vi "PC Code 2.vi"() -> ()   [LabVIEW 2014]
uses:
  <vilib>/Instr/_visa.llb/VISA Flush IO Buffer Mask.ctl
panel:
  in  "stop":bool caption="ESTOP"
  out "String Received":string
  in  "VISA resource name":refnum<visa-resource-name>="COM10"
  in  "error in":errorcluster
  out "Battery\nVolts":i16
  out "Mode":i16=1
  out "Local\nHeading":i16=90
  out "Desired \nVelocity":i16=5
  out "Dist":i16
  out "IR Index":i32
  out "error out":errorcluster
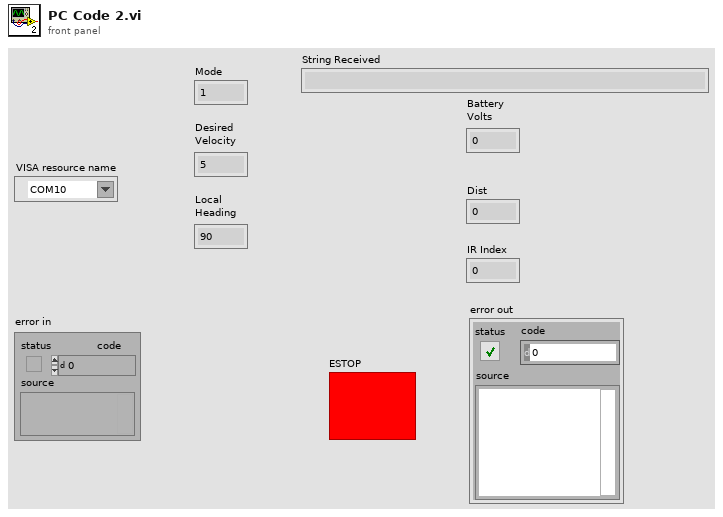
[diagram p1: front panel]
types:
  T1 = typedef "VISA Flush IO Buffer Mask.ctl" = u16
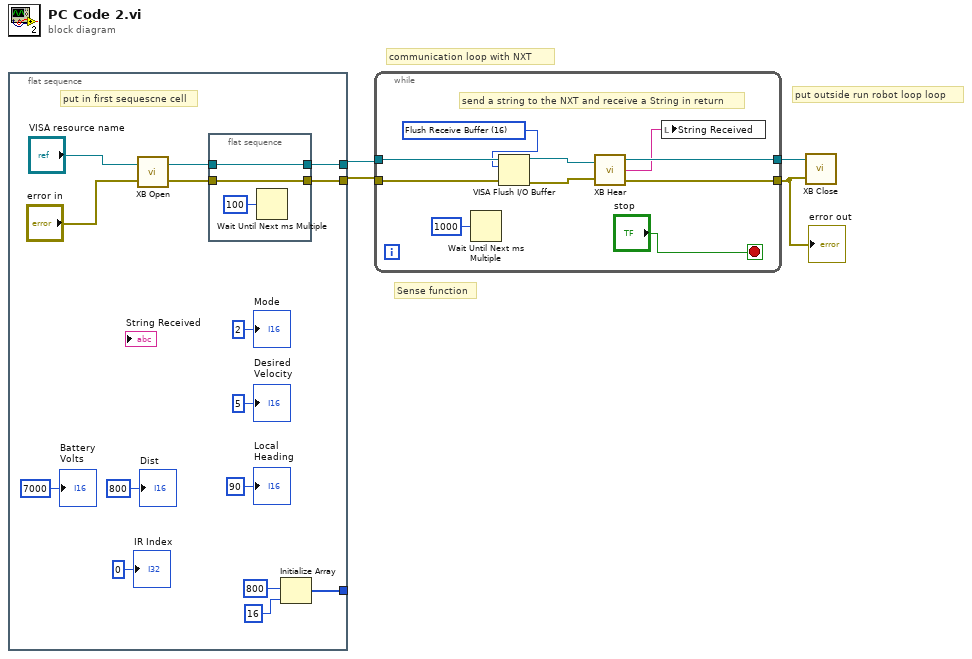
[diagram p0: block diagram]
diagram:
  # "put outside run robot loop loop"
  # "Sense function"
  # "communication loop with NXT"
  n1 = flat-sequence {
    tunnel: [w15] -> w3
    tunnel: [w14] -> w2
    tunnel: [w5] -> _
    frame #0 {
      # "put in first sequescne cell"
      n2 = call "XB Open.vi"("error in (no error)"="error in", "VISA resource name"="VISA resource name") -> ("error out"=w18:errorcluster, "VISA resource name out"=w19:refnum<visa-resource-name>)
      n3 = flat-sequence {
        tunnel: w19 -> [w20]
        tunnel: w18 -> [w21]
        tunnel: [w21] -> w14
        tunnel: [w20] -> w15
        frame #0 {
          n4 = Wait Until Next ms Multiple(millisecond multiple=u32 100) -> ()  [unwired: 1 out]
        }
      }
      n5 = Initialize Array(i16 800, 16 ("dimension size")) -> (w5:i16[])
      "Battery\nVolts" <- i16 7000 ("Battery\nVolts")
      "Mode" <- i16 2 ("Mode")
      "Local\nHeading" <- i16 90 ("Local\nHeading")
      "Desired \nVelocity" <- i16 5 ("Desired \nVelocity")
      "Dist" <- i16 800 ("Dist")
      "IR Index" <- 0 ("IR Index")
    }
  }
  n6 = while {
    tunnel: w3 -> [w25]
    tunnel: w2 -> [w27]
    tunnel: [w32] -> w1
    tunnel: [w31] -> w4
    stop <- "stop" stop-if-true
    w23 = T1 16 items=["Flush Receive Buffer"=16, "Write Transmit Buffer to Device"=32, "Flush Receive Buffer (No I/O)"=64, "Flush Transmit Buffer"=128] ("Mask")
    # "send a string to the NXT and receive a String in return"
    n7 = Wait Until Next ms Multiple(millisecond multiple=u32 1000) -> ()  [unwired: 1 out]
    n8 = VISA Flush I/O Buffer(VISA resource name=w25, mask (16)=w23, error in (no error)=w27) -> (VISA resource name out=w24:refnum<visa-resource-name>, error out=w26:errorcluster)
    n9 = call "XB Hear.vi"("VISA resource name"=w24, "error in (no error)"=w26) -> ("VISA resource name out"=w31:refnum<visa-resource-name>, "String Received"=w29:string, "error out"=w32:errorcluster)
    n10 = local write "String Received"(w29) -> ()
  }
  "error out" <- w1
  n11 = call "XB Close.vi"("error in (no error)"=w1, "VISA resource name"=w4) -> ()
